vi "Build Text Message.vi"(8 "Message Content":string, 9 "Message Tag":string, 10 "Facility Code":T1=enum."user", 11 "Severity Code":T2=enum."error") -> (3 "Syslog Message":string)   [LabVIEW 2021, in "Event_TextLog.lvclass"]
uses:
  Event_TextLog.lvclass
  abs_EventLog/Support/Severity Code.ctl
  abs_EventLog/Support/Facility Code.ctl
  abs_EventLog/abs_EventLog.lvclass
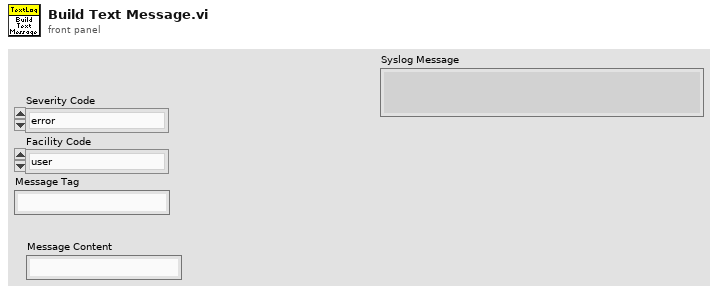
[diagram p1: front panel]
types:
  T1 = typedef "abs_EventLog.lvclass/Facility Code.ctl" = enum16{"kernel", "user", "mail", "system daemons", "security/authorization", "syslogd", "line printer", "network news", "uucp", "clock daemon", "security/authorization (alternate)", "FTP daemon", "NTP subsystem", "log audit", "log alert", "clock daemon (alternate)", "local use 0", "local use 1", "local use 2", "local use 3", "local use 4", "local use 5", "local use 6", "local use 7"}
  T2 = typedef "abs_EventLog.lvclass/Severity Code.ctl" = enum16{"emergency", "alert", "critical", "error", "warning", "notice", "info", "debug"}
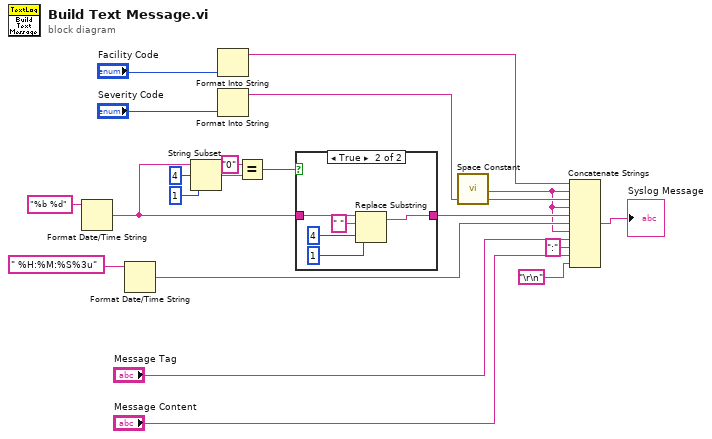
[diagram p0: block diagram]
diagram:
  n1 = Format Date/Time String(time format string (%c)="%b %d") -> (date/time string=w14:string)  [unwired: 2 in]
  n2 = Format Date/Time String(time format string (%c)=" %H:%M:%S%3u") -> (date/time string=w12:string)  [unwired: 2 in]
  n3 = String Subset(string=w14, offset (0)=4, length (rest)=1 ("length (rest)")) -> (substring=w17:string)
  n4 = Format Into String("Facility Code") -> (resulting string=w5:string)  [unwired: 3 in, 1 out]
  n5 = Format Into String("Severity Code") -> (resulting string=w4:string)  [unwired: 3 in, 1 out]
  n6 = Equal?(x="0", y=w17) -> (x = y?=w15:bool)
  n7 = case shown="True" w15 {
    tunnel: w14 -> [w21 w26]
    tunnel: [w21 w22] -> w13
    frame False {
    }
    frame True {
      n8 = Replace Substring(2:1 ("length (len. of substring)"), 3:4 ("offset (0)"), 4:" " ("substring (\"\")"), 5:w26) -> (1:w22:string)  [unwired: 1 out]
    }
  }
  n9 = call <vilib>:"Space Constant.vi"() -> ("String"=w2:string)
  n10 = Concatenate Strings(w5, w2, w4, w2, w13, w12, w2, "Message Tag", ":" ("string"), "Message Content", "\r\n") -> (→"Syslog Message":string)
